vi "gRPC Server.vi"(8 "error in (no error)":errorcluster, 11 "CIFPlugin in":refnum<class "Template_Plugin.lvclass">) -> (0 "error out":errorcluster, 3 "CIFPlugin out":refnum<class "Template_Plugin.lvclass">)   [LabVIEW 2021, in "Template_Plugin.lvclass"]
uses:
  Template_Plugin.lvclass
  Template_Plugin.lvclass/Template_Plugin.ctl
  <vilib>/CIF Foundation/CIF Core/CIFCore/Class/CIFCorePlugin.lvclass
  Grpc/Template_server/RPC Service/Template/Template.lvclass
  Grpc/Template_server/RPC Messages/cif_common_Status.ctl
  Grpc/Template_server/Template_server.lvlib
  C:/Program Files/National Instruments/LabVIEW 2021/vi.lib/CIF Foundation/CIF Core/CIFCore/Class/CIFCorePlugin.lvclass
  Grpc/Template_server/RPC Messages/cif_template_GetStatisticsResponse.ctl
  Grpc/Template_server/RPC Messages/cif_template_SetNumericResponse.ctl
  Grpc/Template_server/RPC Messages/cif_template_GetResultResponse.ctl
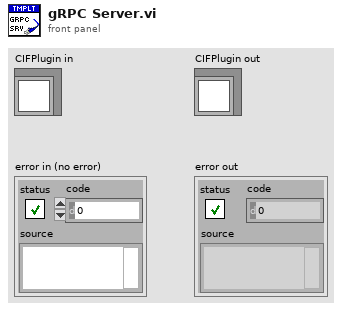
[diagram p1: front panel]
types:
  T1 = typedef "Template_server.lvlib/cif_template_SetNumericResponse.ctl" = cluster{"status":T2}
  T2 = typedef "Template_server.lvlib/cif_common_Status.ctl" = cluster{"code":i32, "message":string}
  T3 = typedef "Template_server.lvlib/cif_template_GetResultResponse.ctl" = cluster{"result":i32}
  T4 = typedef "Template_server.lvlib/cif_template_GetStatisticsResponse.ctl" = cluster{"iterations":u64}
  T5 = typedef "grpc-lvsupport-release.lvlib/grpcId.ctl" = u64
  T6 = typedef "Template_server.lvlib/cif_template_SetNumericRequest.ctl" = cluster{"numeric":i32}
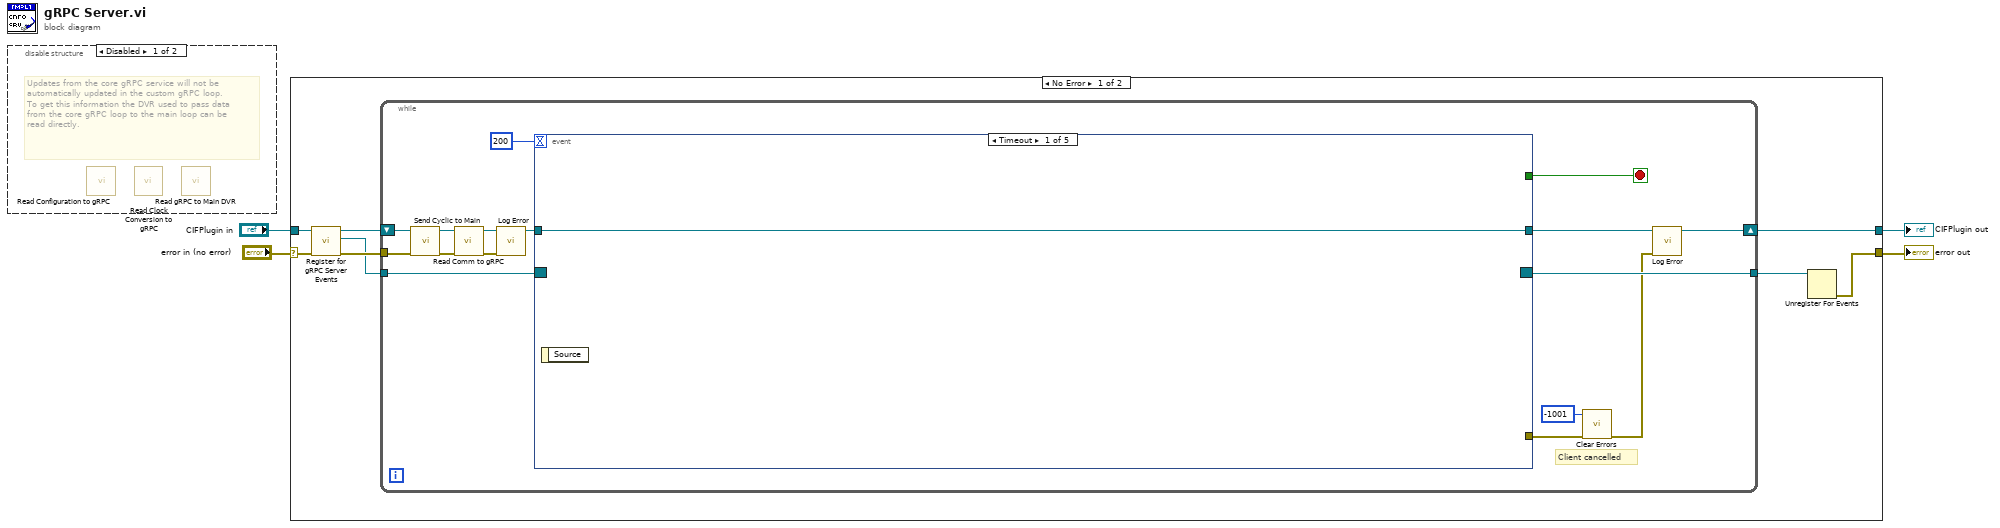
[diagram p0: block diagram]
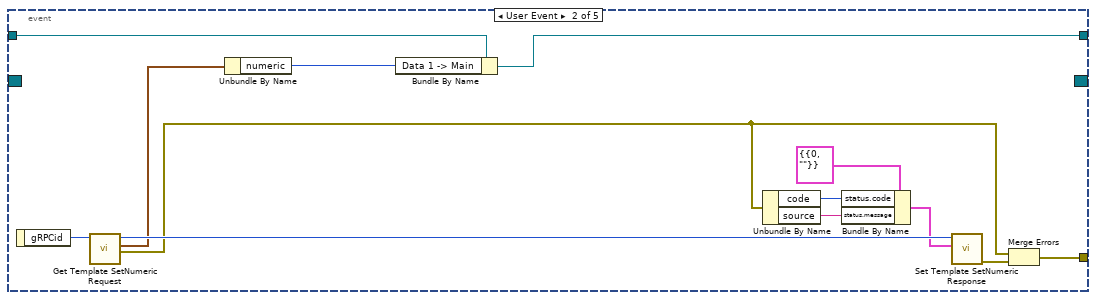
[diagram p3: hidden frame]
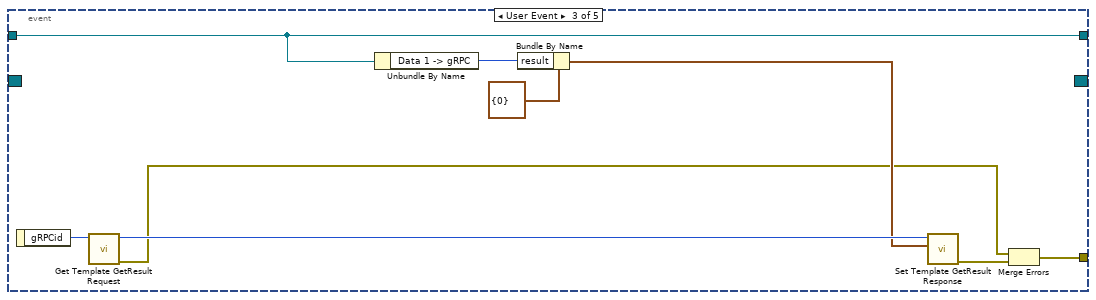
[diagram p4: hidden frame]
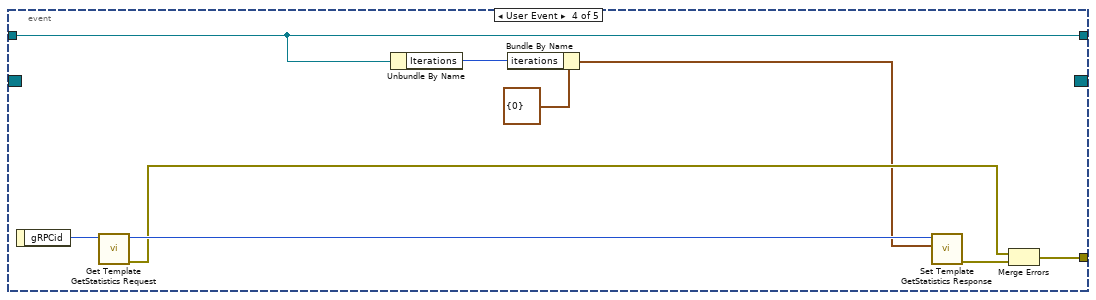
[diagram p5: hidden frame]
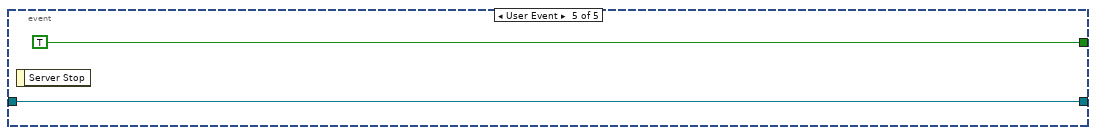
[diagram p6: hidden frame]
diagram:
  n1 = disable-structure shown="Disabled" {
    frame Disabled {
      # "Updates from the core gRPC service will not be automatically updated in the custom gRPC loop.  To get this information the DVR used to pass data from the core gRPC loop to the main loop can be read directly."
      n2 = call "Read Configuration to gRPC.vi"() -> ()  [unwired: 9 in, 3 out]
      n3 = call <vilib>:"Read Clock Conversion to gRPC.vi"() -> ()  [unwired: 9 in, 3 out]
      n4 = call <vilib>:"Read gRPC to Main DVR.vi"() -> ()  [unwired: 9 in, 3 out]
    }
    frame Enabled {
    }
  }
  n5 = case shown="No Error" "error in (no error)" {
    selector: "error in (no error)" -> [w9 w63]
    tunnel: "CIFPlugin in" -> [w10 w64]
    tunnel: [w11 w64] -> w3
    tunnel: [w6 w63] -> w4
    frame No Error {
      n6 = call "Register for gRPC Server Events.vi"("error in (no error)"=w9, "CIFPlugin in"=w10) -> ("error out"=w8:errorcluster, "Event Registration Refnum"=w5:refnum<event-registration>, "CIFPlugin out"=w7:refnum<class "Template_Plugin.lvclass">)  [unwired: 7 in]
      n7 = while {
        tunnel: w5 -> [w13]
        tunnel: w8 -> [w21]
        tunnel: [w26] -> w12
        shift-right: [w24] -> w11
        shift-left: w7 -> [w22]
        stop <- w27 stop-if-true
        # "Client cancelled"
        n8 = call "Send Cyclic to Main.vi"("error in (no error)"=w21, "CIFPlugin in"=w22) -> ("error out"=w19:errorcluster, "CIFPlugin out"=w20:refnum<class "Template_Plugin.lvclass">)  [unwired: 8 in]
        n9 = call "Read Comm to gRPC.vi"("error in (no error)"=w19, "CIFPlugin in"=w20) -> ("error out"=w17:errorcluster, "CIFPlugin out"=w18:refnum<class "Template_Plugin.lvclass">)  [unwired: 8 in]
        n10 = call <vilib>:"Log Error.vi"("error in (no error)"=w17, "CIFCorePlugin in"=w18) -> ("CIFCorePlugin out"=w23:refnum<class "Template_Plugin.lvclass">)  [unwired: 8 in, 1 out]
        n11 = event shown="[0] Timeout" {
          selector: w13 -> [_ _ _ _ _]
          dyn-events: [_ _ _ _ _] -> w26
          timeout: 200 -> [_ _ _ _ _]
          tunnel: w23 -> [w29 w35 w50 w59 w61]
          tunnel: [_ w40 w51 w60 _] -> w15
          tunnel: [w29 w33 w50 w59 w61] -> w25
          tunnel: [_ _ _ _ TRUE] -> w27
          event Timeout {
            n12 = event-data() -> ()  [unwired: 1 in, 1 out]
          }
          event User Event {
            n13 = event-data() -> ("gRPCid"=w38:T5)  [unwired: 1 in]
            n14 = call "Get Template SetNumeric Request.vi"("gRPCid"=w38) -> ("error out"=w32:errorcluster, "Message Data"=w36:T6, "gRPCid out"=w39:T5)  [unwired: 8 in]
            n15 = Unbundle By Name(w36) -> ("numeric"=w34:i32)
            n16 = Bundle By Name(cluster=w35, "Data 1 -> Main"=w34) -> (w33:refnum<class "Template_Plugin.lvclass">)
            n17 = Unbundle By Name(w32) -> ("code"=w42:i32, "source"=w41:string)
            n18 = Bundle By Name(cluster=T1 {"status"={"code"=0, "message"=""}} ("Message Data"), "status.code"=w42, "status.message"=w41) -> (w30:T1)
            n19 = call "Set Template SetNumeric Response.vi"("Message Data"=w30, "gRPCid in"=w39) -> ("error out"=w37:errorcluster)  [unwired: 9 in]
            n20 = Merge Errors(w32, w37) -> (w40:errorcluster)
          }
          event User Event {
            n21 = event-data() -> ("gRPCid"=w48:T5)  [unwired: 1 in]
            n22 = call "Get Template GetResult Request.vi"("gRPCid"=w48) -> ("error out"=w45:errorcluster, "gRPCid out"=w47:T5)  [unwired: 8 in, 1 out]
            n23 = Unbundle By Name(w50) -> ("Data 1 -> gRPC"=w49:i32)
            n24 = Bundle By Name(cluster=T3 {"result"=0} ("Message Data"), "result"=w49) -> (w46:T3)
            n25 = call "Set Template GetResult Response.vi"("Message Data"=w46, "gRPCid in"=w47) -> ("error out"=w44:errorcluster)  [unwired: 9 in]
            n26 = Merge Errors(w45, w44) -> (w51:errorcluster)
          }
          event User Event {
            n27 = event-data() -> ("gRPCid"=w57:T5)  [unwired: 1 in]
            n28 = call "Get Template GetStatistics Request.vi"("gRPCid"=w57) -> ("error out"=w54:errorcluster, "gRPCid out"=w56:T5)  [unwired: 8 in, 1 out]
            n29 = Unbundle By Name(w59) -> ("Iterations"=w58:u64)
            n30 = Bundle By Name(cluster=T4 {"iterations"=0} ("Message Data"), "iterations"=w58) -> (w53:T4)
            n31 = call "Set Template GetStatistics Response.vi"("Message Data"=w53, "gRPCid in"=w56) -> ("error out"=w55:errorcluster)  [unwired: 9 in]
            n32 = Merge Errors(w54, w55) -> (w60:errorcluster)
          }
          event User Event {
            n33 = event-data() -> ()  [unwired: 1 in, 1 out]
          }
        }
        n34 = call <vilib>:"Clear Errors.vi"("error in (no error)"=w15, "specific error code to clear (0: all)"=-1001) -> ("error out"=w14:errorcluster)  [unwired: 4 in, 1 out]
        n35 = call <vilib>:"Log Error.vi"("error in (no error)"=w14, "CIFCorePlugin in"=w25) -> ("CIFCorePlugin out"=w24:refnum<class "Template_Plugin.lvclass">)  [unwired: 8 in, 1 out]
      }
      n36 = Unregister For Events(event registration refnum=w12) -> (error out=w6:errorcluster)  [unwired: 1 in]
    }
    frame Error {
    }
  }
  "error out" <- w4
  "CIFPlugin out" <- w3
